vi "get channels.vi"(11 "Sequencer Module configuration in":refnum<class "Sequencer Module configuration.lvclass">) -> (2 "channels":refnum<class "TBM channel.lvclass">[](array[class]), 3 "Sequencer Module configuration out":refnum<class "Sequencer Module configuration.lvclass">)   [LabVIEW 2015, in "Sequencer Module configuration.lvclass"]
doc: "Returns an array of all Channels currently added to this configuration object."
uses:
  Sequencer Module configuration.lvclass
  <vilib>/NI/Tag Bus Module Framework/channel/TBM channel.lvclass
  Sequencer Module configuration.lvclass/Sequencer Module configuration.ctl
  <vilib>/NI/Tag Bus/tag/tag descriptor.lvclass/tag descriptor.ctl
  <vilib>/NI/Tag Bus/tag/read tag name.vi
  <vilib>/NI/Tag Bus/tag/tag descriptor.lvclass
  classes/Sequence Config/Sequence Config.lvclass
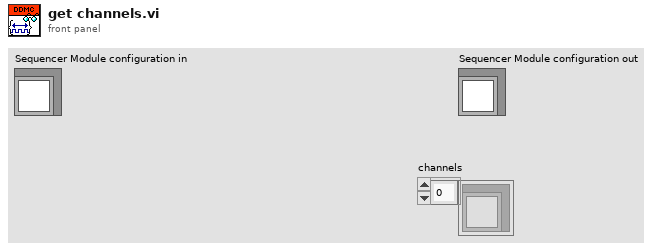
[diagram p1: front panel]
types:
  T1 = typedef "Sequencer Module configuration.lvclass/Line.ctl" = cluster{"Sequence":refnum<class "Sequence Config.lvclass">}
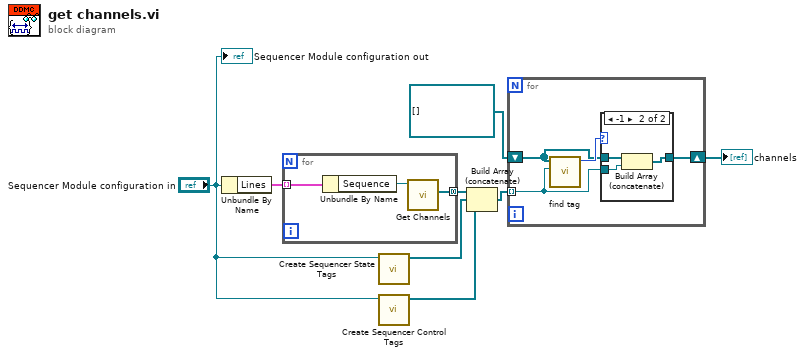
[diagram p0: block diagram]
diagram:
  n1 = Unbundle By Name("Sequencer Module configuration in") -> ("Lines"=w8:T1[])
  n2 = for {
    tunnel: w8 -> [w11] mode=indexing
    tunnel: [w9] -> w6 mode=concatenating
    n3 = Unbundle By Name(w11) -> ("Sequence"=w10:refnum<class "Sequence Config.lvclass">)
    n4 = call "Get Channels.vi"("Sequence Config in"=w10) -> ("Channels"=w9:refnum<class "TBM channel.lvclass">[])  [unwired: 8 in, 2 out]
  }
  n5 = call "Create Sequencer State Tags.vi"("Sequencer Module configuration in"="Sequencer Module configuration in") -> ("Array"=w3:refnum<class "TBM channel.lvclass">[])  [unwired: 10 in]
  n6 = call "Create Sequencer Control Tags.vi"("Sequencer Module configuration in"="Sequencer Module configuration in") -> ("Array"=w1:refnum<class "TBM channel.lvclass">[])  [unwired: 10 in]
  n7 = Build Array (concatenate)(w6, w3, w1) -> (w4:refnum<class "TBM channel.lvclass">[])
  n8 = for {
    tunnel: w4 -> [w12] mode=indexing
    shift-right: [w14] -> w5
    shift-left: refnum<class "TBM channel.lvclass">[] [] ("Channels") -> [w13]
    n9 = call <vilib>:"find tag.vi"("tag"=w12, "tags in"=w13) -> ("index"=w15:i32)  [unwired: 9 in]
    n10 = case shown="-1" w15 {
      tunnel: [w16 w17] -> w14
      tunnel: w13 -> [w16 w19]
      tunnel: w12 -> [_ w18]
      frame 0, Default {
      }
      frame -1 {
        n11 = Build Array (concatenate)(w19, w18) -> (w17:refnum<class "TBM channel.lvclass">[])
      }
    }
  }
  "channels" <- w5
  "Sequencer Module configuration out" <- "Sequencer Module configuration in"
